vi "GLOBAL Debug.vi"() -> ()   [LabVIEW 2016]
panel:
  in  "String":string
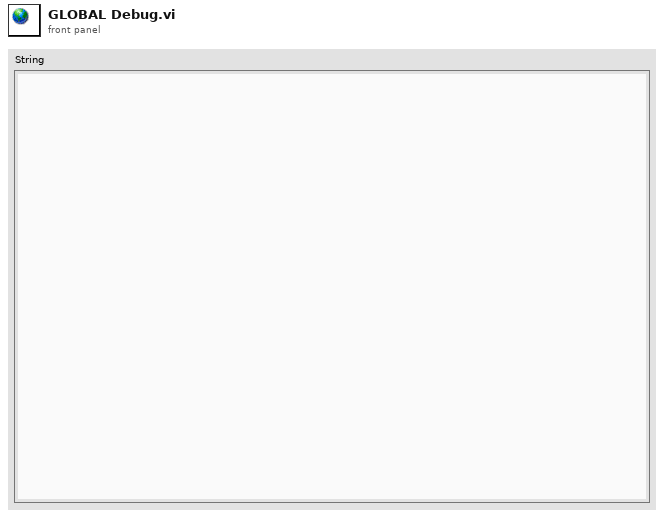
[diagram p1: front panel]
diagram:
